vi "Initialize.vi"(8 "error in (no error)":errorcluster, 10 "config path":path, 11 "Lamp in":refnum<class "Lamp.lvclass">) -> (0 "error out":errorcluster, 3 "Lamp out":refnum<class "Lamp.lvclass">)   [LabVIEW 2016, in "Lamp.lvclass"]
uses:
  Lamp.lvclass
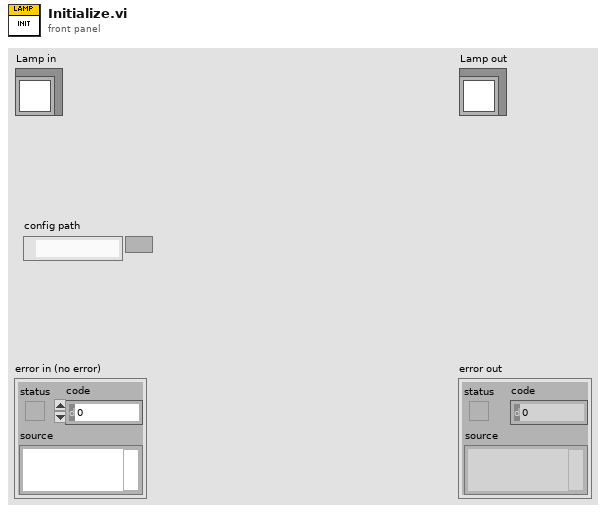
[diagram p1: front panel]
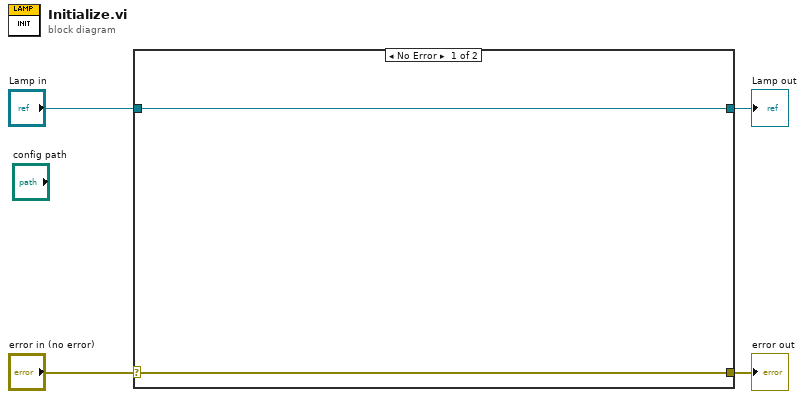
[diagram p0: block diagram]
diagram:
  n1 = case shown="No Error" "error in (no error)" {
    selector: "error in (no error)" -> [w5 w8]
    tunnel: [w5 w8] -> w3
    tunnel: [w6 w7] -> w1
    tunnel: "Lamp in" -> [w6 w7]
    frame No Error {
    }
    frame Error {
    }
  }
  "error out" <- w3
  "Lamp out" <- w1
